vi "Equal.vi"() -> ()   [LabVIEW 2017, in "Assertions.Tests.lvlib" / "Assert Greater Than.lvlib"]
uses:
  Assert Greater Than.lvlib
  6f85d698-f017-4718-9ab7-7a02d42b0a52.vi
  src/Transparent Assertions/Constraints/Is Greater Than/Create.vi
  src/Transparent Assertions/Constraints/Is Greater Than/Is Greater Than.lvclass
  src/Transparent Assertions/Assertions/Assertions.lvlib
panel:
  out "error out":errorcluster
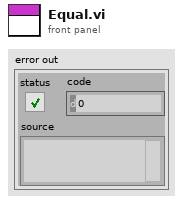
[diagram p1: front panel]
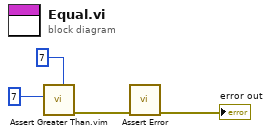
[diagram p0: block diagram]
diagram:
  n1 = call "Assert Greater Than.vim"("Expected"=7, "Actual"=7) -> ("error out"=w4:errorcluster)  [unwired: 9 in]
  n2 = call "Assert Error.vi"("error in (no error)"=w4) -> ("error out"=→"error out":errorcluster)  [unwired: 10 in]
